vi "FlatToRichcif_manager_QueryClockStatusResponse.vi"(5 "OutputClusterType":T1, 11 "InputCluster":T6) -> (3 "OutputCluster":T1)   [LabVIEW 2021, in "CIF_Manager_client.lvlib"]
uses:
  CIF_Manager_client.lvlib
  cif_manager_QueryClockStatusResponse_Flat.ctl
  cif_manager_ClockStatusArray_Flat.ctl
  cif_manager_ClockStatus_Flat.ctl
  cif_manager_ClockConversion_Flat.ctl
  cif_manager_TimePair_Flat.ctl
  cif_manager_QueryClockStatusResponse.ctl
  cif_manager_ClockStatusArray.ctl
  cif_manager_ClockStatus.ctl
  cif_manager_ClockConversion.ctl
  cif_manager_TimePair.ctl
  FlatToRichcif_manager_ClockStatus.vi
  FlatToRichcif_manager_ClockConversion.vi
  FlatToRichcif_manager_TimePair.vi
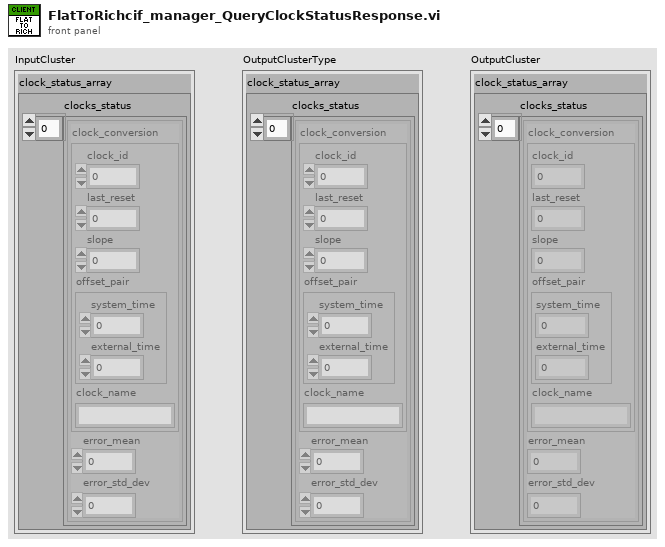
[diagram p1: front panel]
types:
  T1 = typedef "CIF_Manager_client.lvlib/cif_manager_QueryClockStatusResponse.ctl" = cluster{"clock_status_array":T2}
  T2 = typedef "CIF_Manager_client.lvlib/cif_manager_ClockStatusArray.ctl" = cluster{"clocks_status":T3[]}
  T3 = typedef "CIF_Manager_client.lvlib/cif_manager_ClockStatus.ctl" = cluster{"clock_conversion":T4, "error_mean":i64, "error_std_dev":i64}
  T4 = typedef "CIF_Manager_client.lvlib/cif_manager_ClockConversion.ctl" = cluster{"clock_id":u32, "last_reset":i64, "slope":dbl, "offset_pair":T5, "clock_name":string}
  T5 = typedef "CIF_Manager_client.lvlib/cif_manager_TimePair.ctl" = cluster{"system_time":i64, "external_time":i64}
  T6 = typedef "CIF_Manager_client.lvlib/cif_manager_QueryClockStatusResponse_Flat.ctl" = cluster{"clock_status_array":T7}
  T7 = typedef "CIF_Manager_client.lvlib/cif_manager_ClockStatusArray_Flat.ctl" = cluster{"clocks_status":T8[]}
  T8 = typedef "CIF_Manager_client.lvlib/cif_manager_ClockStatus_Flat.ctl" = cluster{"clock_conversion":T9, "error_mean":i64, "error_std_dev":i64}
  T9 = typedef "CIF_Manager_client.lvlib/cif_manager_ClockConversion_Flat.ctl" = cluster{"clock_id":u32, "last_reset":i64, "slope":dbl, "offset_pair":T10, "clock_name":string}
  T10 = typedef "CIF_Manager_client.lvlib/cif_manager_TimePair_Flat.ctl" = cluster{"system_time":i64, "external_time":i64}
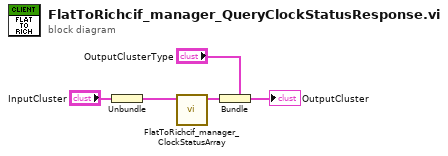
[diagram p0: block diagram]
diagram:
  n1 = Unbundle "Unbundle"("InputCluster") -> ("clock_status_array"=w2:T7)
  n2 = call "FlatToRichcif_manager_ClockStatusArray.vi"("InputCluster"=w2) -> ("OutputCluster"=w1:T2)  [unwired: 10 in]
  n3 = Bundle "Bundle"(cluster="OutputClusterType", "clock_status_array"=w1) -> (→"OutputCluster":T1)
